vi "Database-DecodePageID.vi"(11 "PageID":string) -> (3 "Decoded Page ID":string)   [LabVIEW 2013]
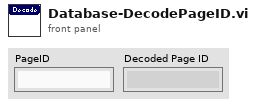
[diagram p1: front panel]
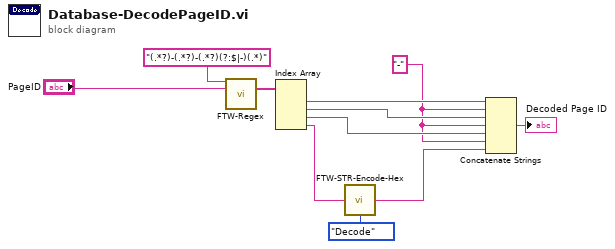
[diagram p0: block diagram]
diagram:
  w3 = "-" ("string")
  n1 = call "FTW-Regex.vi"("Regular Expression"="(.*?)-(.*?)-(.*?)(?:$|-)(.*)" ("regular expression"), "Input String"="PageID") -> ("Submatches"=w10:string[])  [unwired: 9 in, 4 out]
  n2 = Index Array(array=w10) -> (element #1=w6:string, element #2=w5:string, element #3=w4:string, element #4=w8:string)  [unwired: 4 in]
  n3 = call "FTW-STR-Encode-Hex.vi"("Input"=w8, "Direction"=enum16{"Encode", "Decode"}."Decode") -> ("Output"=w2:string)
  n4 = Concatenate Strings(w6, w3, w5, w3, w4, w3, w2) -> (→"Decoded Page ID":string)
